vi "Execute.vi"(8 "error in (no error)":errorcluster, 11 "Order In":refnum<class "Order.lvclass">) -> (0 "error out":errorcluster, 3 "Order Out":refnum<class "Order.lvclass">)   [LabVIEW 2019, in "Order.lvclass"]
doc: "Execute must be overriden by child classes."
uses:
  Order.lvclass
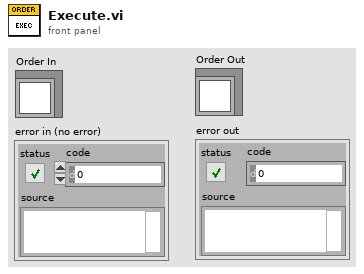
[diagram p1: front panel]
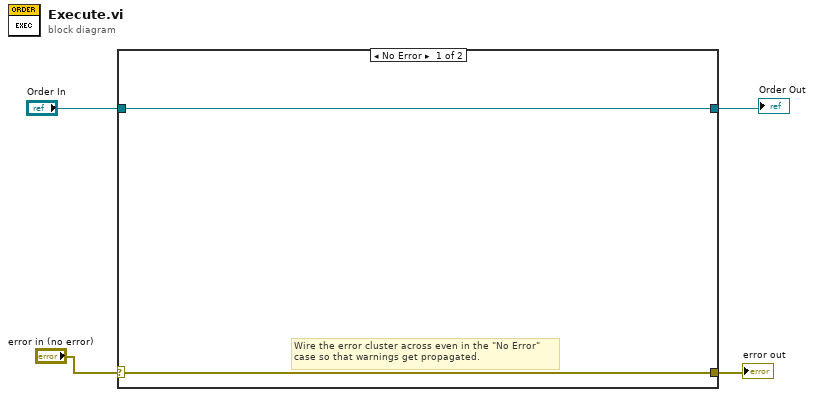
[diagram p0: block diagram]
diagram:
  n1 = case shown="No Error" "error in (no error)" {
    selector: "error in (no error)" -> [w5 w8]
    tunnel: [w5 w8] -> w1
    tunnel: [w6 w7] -> w4
    tunnel: "Order In" -> [w6 w7]
    frame No Error {
      # "Wire the error cluster across even in the \"No Error\"\ncase so that warnings get propagated."
    }
    frame Error {
      # "The order doesn't have any functionality here\nMust be overridden"
    }
  }
  "error out" <- w1
  "Order Out" <- w4
